vi "MSEncoder SubVI WfmCodeGen_OutputWfm.vi"(8 "error in (no error)":errorcluster, 11 "calc wfm queue":refnum<queue>) -> (0 "error out":errorcluster, 3 "WfmCode":u64[](array[numeric]))   [LabVIEW 2018, in "MSEncoder.lvclass"]
uses:
  MSEncoder.lvclass
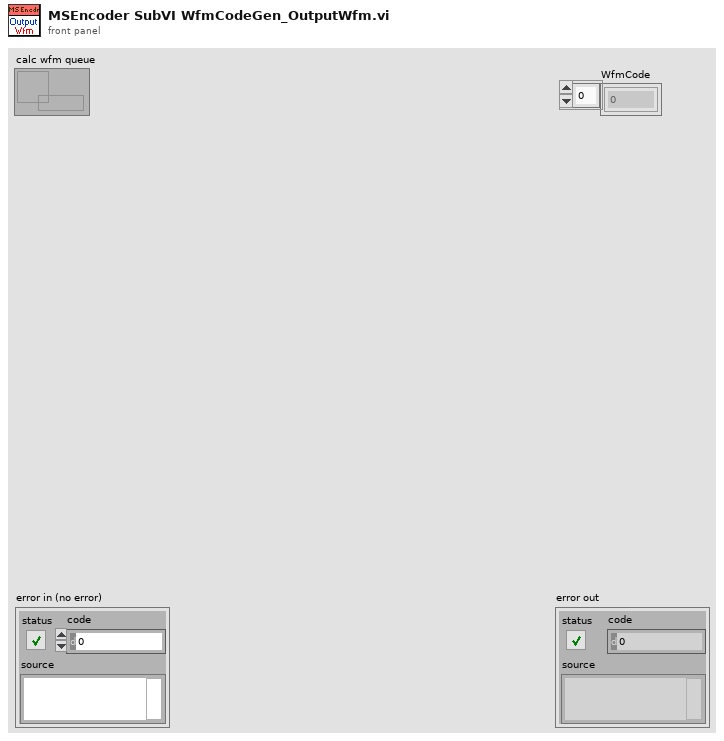
[diagram p1: front panel]
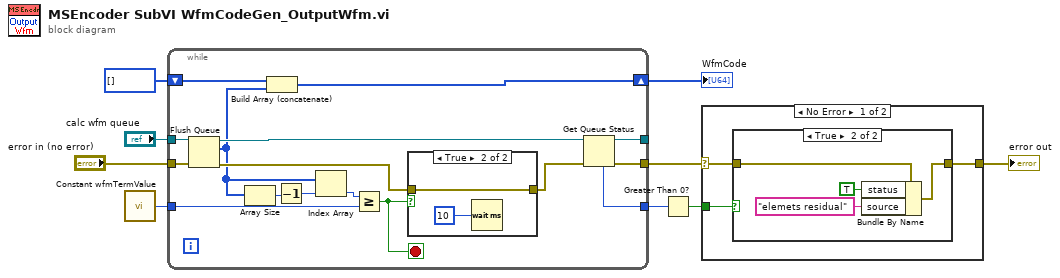
[diagram p0: block diagram]
diagram:
  n1 = call "Constant wfmTermValue.vi"() -> ("wfm end value"=w6:u64)
  n2 = while {
    tunnel: "calc wfm queue" -> [w17]
    tunnel: "error in (no error)" -> [w15]
    tunnel: [w20] -> _
    tunnel: [w19] -> w3
    shift-right: [w25] -> w5
    shift-left: u64[] [] -> [w24]
    tunnel: w6 -> [w23]
    tunnel: [w18] -> w4
    stop <- w22 stop-if-true
    n3 = Flush Queue(queue=w17, error in (no error)=w15) -> (queue out=w16:refnum<queue>, remaining elements=w12:u64[], error out=w14:errorcluster)
    n4 = Array Size(array=w12) -> (size(s)=w10:i32)
    n5 = Build Array (concatenate)(w24, w12) -> (w25:u64[])
    n6 = Decrement(x=w10) -> (x-1=w11:i32)
    n7 = Index Array(array=w12, index=w11) -> (element=w13:u64)
    n8 = Greater Or Equal?(x=w13, y=w23) -> (x >= y?=w22:bool)
    n9 = case shown="True" w22 {
      tunnel: w14 -> [w26 w27]
      tunnel: [w26 w27] -> w21
      frame False {
      }
      frame True {
        n10 = Wait (ms)(milliseconds to wait=u32 10) -> ()  [unwired: 1 out]
      }
    }
    n11 = Get Queue Status(queue=w16, error in (no error)=w21) -> (queue out=w20:refnum<queue>, error out=w19:errorcluster, # elements in queue=w18:i32)  [unwired: 1 in, 5 out]
  }
  "WfmCode" <- w5
  n12 = Greater Than 0?(x=w4) -> (x > 0?=w2:bool)
  n13 = case shown="No Error" w3 {
    selector: w3 -> [w30 w37]
    tunnel: w2 -> [w31 _]
    tunnel: [w29 w37] -> w1
    frame No Error {
      n14 = case shown="True" w31 {
        tunnel: w30 -> [w32 w36]
        tunnel: [w32 w33] -> w29
        frame False {
        }
        frame True {
          n15 = Bundle By Name(cluster=w36, "status"=TRUE, "source"="elemets residual") -> (w33:errorcluster)
        }
      }
    }
    frame Error {
    }
  }
  "error out" <- w1
